vi "ReadTrace.vi"(8 "error in (no error)":errorcluster, 11 "Instrument in":refnum<class "Instrument.lvclass">) -> (0 "error out":errorcluster, 2 "Trace Spectrum":T1(graph), 3 "Instrument out":refnum<class "Instrument.lvclass">)   [LabVIEW 2014, in "Instrument.lvclass"]
uses:
  Instrument.lvclass
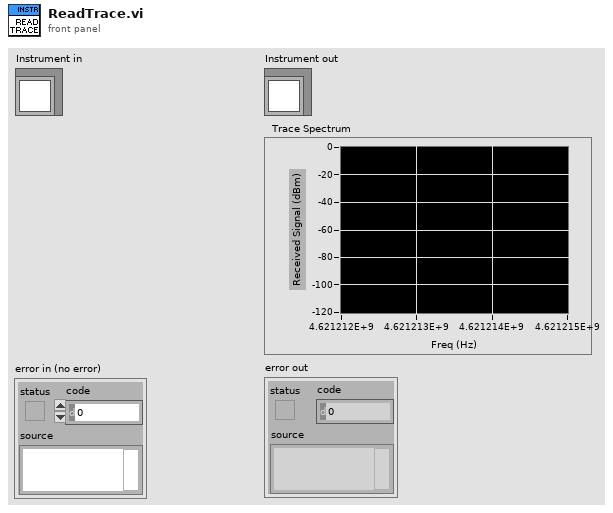
[diagram p1: front panel]
types:
  T1 = cluster{"Initial X":dbl, "X Increment":dbl, "Trace Array":dbl[]}
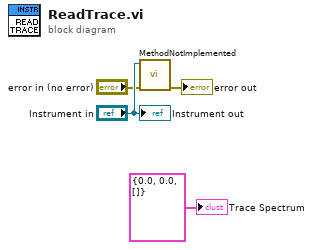
[diagram p0: block diagram]
diagram:
  n1 = call "MethodNotImplemented.vi"("error in (no error)"="error in (no error)", "LabVIEW Object In"="Instrument in") -> ("error out"=→"error out":errorcluster)  [unwired: 9 in]
  "Instrument out" <- "Instrument in"
  "Trace Spectrum" <- T1 {"Initial X"=0.0, "X Increment"=0.0, "Trace Array"=[]} ("Trace Waveform")
